vi "update.vi"(8 "error in (no error)":errorcluster, 11 "DomeController in":refnum<class "DomeController.lvclass">) -> (0 "error out":errorcluster, 3 "DomeController out":refnum<class "DomeController.lvclass">)   [LabVIEW 2016, in "DomeController.lvclass"]
uses:
  DomeController.lvclass
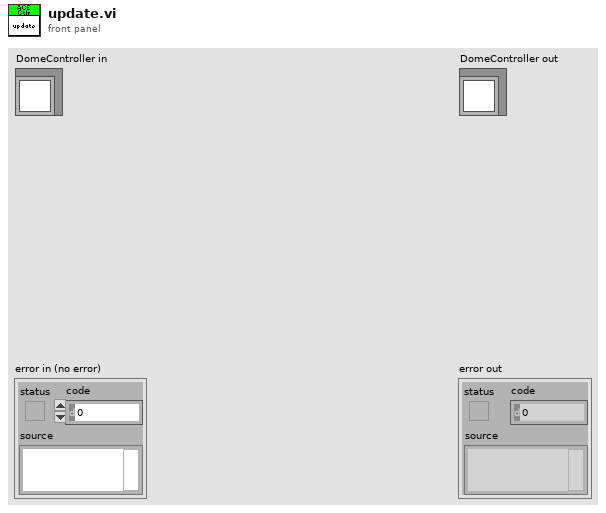
[diagram p1: front panel]
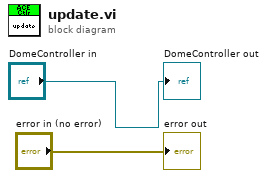
[diagram p0: block diagram]
diagram:
  "error out" <- "error in (no error)"
  "DomeController out" <- "DomeController in"
